vi "KillAllOpenCMD.vi"(8 "error in (no error)":errorcluster) -> (0 "error out":errorcluster)   [LabVIEW 2019]
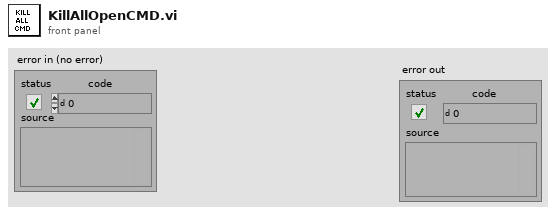
[diagram p1: front panel]
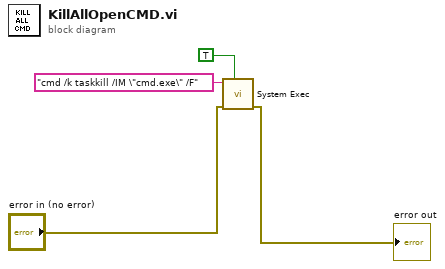
[diagram p0: block diagram]
diagram:
  n1 = call <vilib>:"System Exec.vi"("wait until completion? (T)"=TRUE, "error in (no error)"="error in (no error)", "command line"="cmd /k taskkill /IM \"cmd.exe\" /F") -> ("error out"=→"error out":errorcluster)  [unwired: 5 in, 3 out]
